vi "writeTrigXML.vi"(8 "error in (no error)":errorcluster, 10 "NativeXML in":refnum<class "NativeXML.lvclass">, 11 "WinX32Settings in":refnum<class "WinX32Settings.lvclass">) -> (0 "error out":errorcluster, 2 "NativeXML out":refnum<class "NativeXML.lvclass">, 3 "WinX32Settings out":refnum<class "WinX32Settings.lvclass">)   [LabVIEW 2011, in "Tools.lvlib" / "Settings.lvlib" / "WinX32Settings.lvclass"]
uses:
  WinX32Settings.lvclass
  NativeXML/NativeXML.lvclass
  WinX32Settings.lvclass/WinX32Settings.ctl
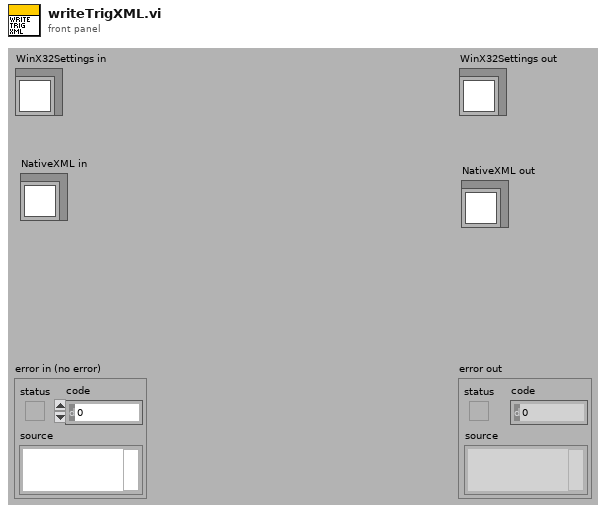
[diagram p1: front panel]
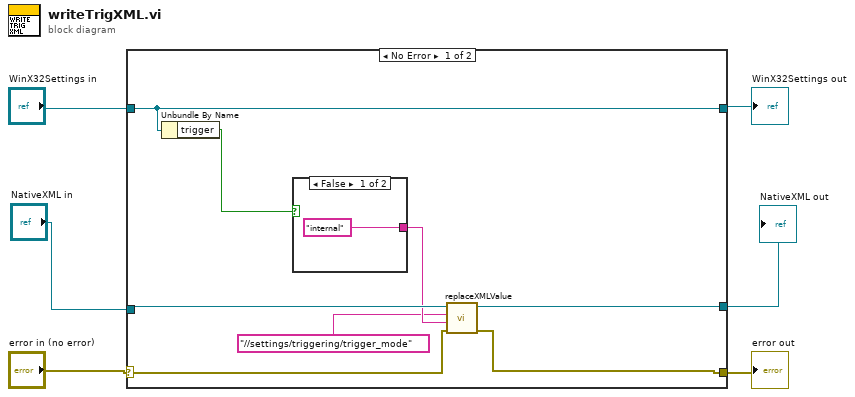
[diagram p0: block diagram]
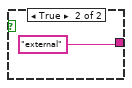
[diagram p2: hidden frame]
diagram:
  n1 = case shown="No Error" "error in (no error)" {
    selector: "error in (no error)" -> [w8 w19]
    tunnel: [w7 w19] -> w3
    tunnel: [w14 w18] -> w1
    tunnel: "WinX32Settings in" -> [w14 w18]
    tunnel: "NativeXML in" -> [w12 w17]
    tunnel: [w11 w17] -> w4
    frame No Error {
      n2 = Unbundle By Name(w14) -> ("trigger"=w13:bool)
      n3 = case shown="False" w13 {
        tunnel: ["internal" "external"] -> w10
        frame False {
        }
        frame True {
        }
      }
      n4 = call "replaceXMLValue.vi"("error in (no error)"=w8, "value"=w10, "replace in"="//settings/triggering/trigger_mode", "NativeXML in"=w12) -> ("error out"=w7:errorcluster, "NativeXML out"=w11:refnum<class "NativeXML.lvclass">)  [unwired: 6 in]
    }
    frame Error {
    }
  }
  "error out" <- w3
  "WinX32Settings out" <- w1
  "NativeXML out" <- w4
